vi "7.2-Joystick Server.vi"() -> ()   [LabVIEW 2010]
doc: "Creates a named service and listens on the first available port. Whenever a client connects to the service, it responds with a message containing joystick data. The VI can be stopped using the STOP button."
uses:
  6-OCU Neurons/6.1-UDP Saitek.ctl
  <vilib>/Utility/inputDevices.llb/joystickAcquire.vi
panel:
  out "direction info":T1
  out "button info":T2
  out "axis info":T3
  out "Saitek Controler":T4 {"Right" scale=-32767.0..32767.0; "Left" scale=-32767.0..32767.0; "Yaw" scale=-32767.0..32767.0; "Roll" scale=-32767.0..32767.0; "Pitch" scale=-32767.0..32767.0}
  out "data out":string
  in  "stop":bool
  out "error out":errorcluster
  in  "error in":errorcluster
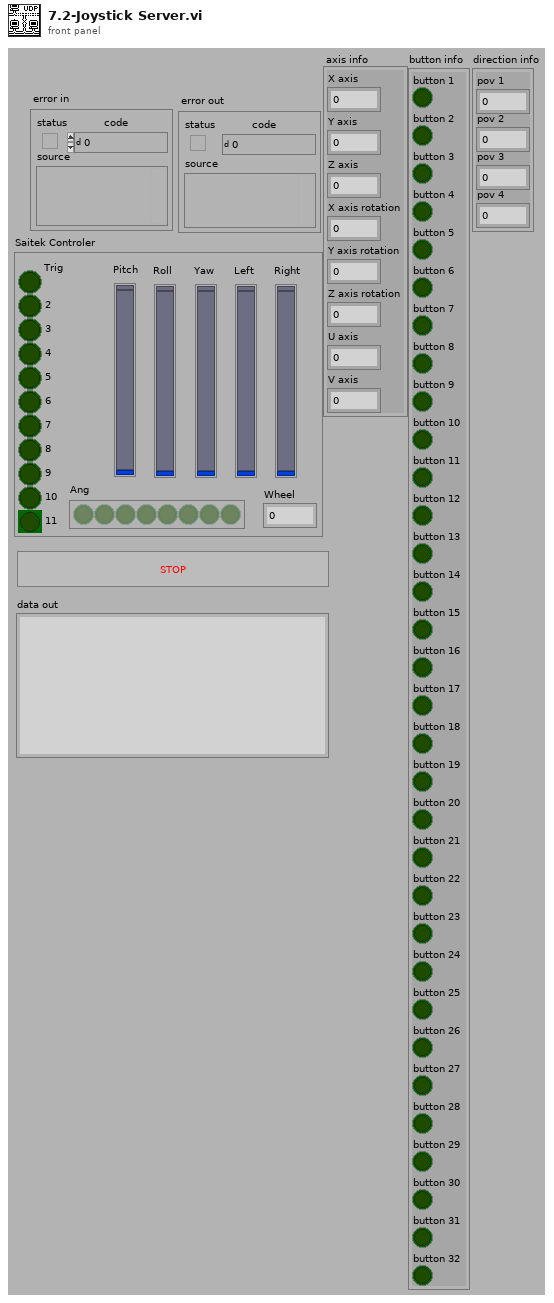
[diagram p1: front panel]
types:
  T1 = cluster{"pov 1":i32, "pov 2":i32, "pov 3":i32, "pov 4":i32}
  T2 = cluster{"button 1":bool, "button 2":bool, "button 3":bool, "button 4":bool, "button 5":bool, "button 6":bool, "button 7":bool, "button 8":bool, "button 9":bool, "button 10":bool, "button 11":bool, "button 12":bool, "button 13":bool, "button 14":bool, "button 15":bool, "button 16":bool, "button 17":bool, "button 18":bool, "button 19":bool, "button 20":bool, "button 21":bool, "button 22":bool, "button 23":bool, "button 24":bool, "button 25":bool, "button 26":bool, "button 27":bool, "button 28":bool, "button 29":bool, "button 30":bool, "button 31":bool, "button 32":bool}
  T3 = cluster{"X axis":i32, "Y axis":i32, "Z axis":i32, "X axis rotation":i32, "Y axis rotation":i32, "Z axis rotation":i32, "U axis":i32, "V axis":i32}
  T4 = typedef "6.1-UDP Saitek.ctl" = cluster{"Trig":bool, "2":bool, "3":bool, "4":bool, "5":bool, "6":bool, "7":bool, "8":bool, "9":bool, "10":bool, "11":bool, "Pitch":i32, "Ang":bool[], "Wheel":dbl, "Roll":i32, "Yaw":i32, "Left":i32, "Right":i32}
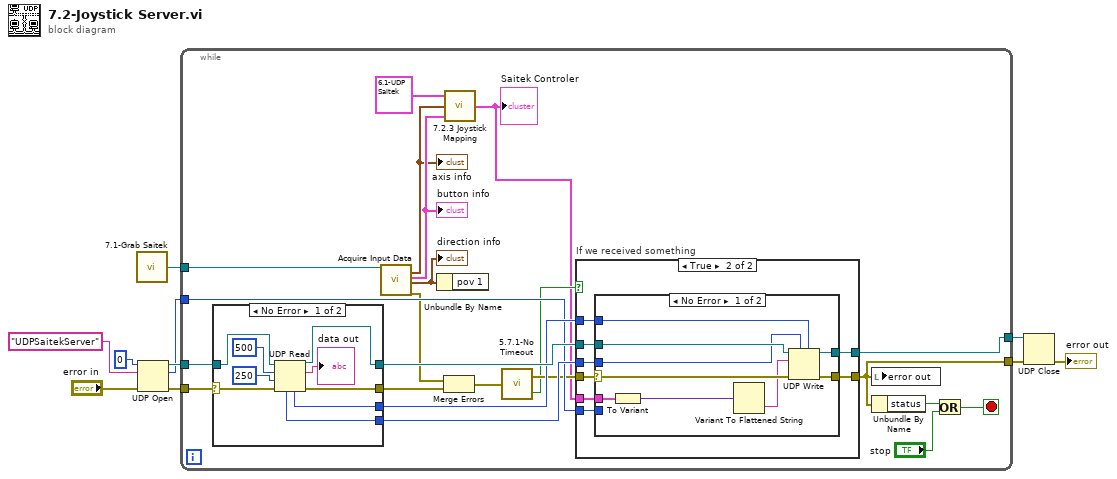
[diagram p0: block diagram]
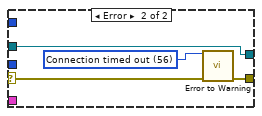
[diagram p3: hidden frame]
diagram:
  n1 = call "7.1-Grab Saitek.vi"() -> ("Saitek ID"=w1:refnum<k1>)
  n2 = UDP Open(8:"error in", 10:"UDPSaitekServer", 11:0) -> (port=w8:refnum<k16>, 0:w7:errorcluster, 2:w3:u16)  [unwired: 2 in]
  n3 = while {
    tunnel: [w20] -> w5
    tunnel: w8 -> [w32]
    tunnel: w7 -> [w29]
    tunnel: [w30] -> w6
    tunnel: w3 -> [w26]
    tunnel: w1 -> [w19]
    stop <- w24 stop-if-true
    n4 = case shown="No Error" w29 {
      selector: w29 -> [w62 w65]
      tunnel: w32 -> [w64 w66]
      tunnel: [w61 w66] -> w31
      tunnel: [w60 w65] -> w18
      tunnel: [w58 _] -> w27
      tunnel: [w59 _] -> w28
      frame No Error {
        n5 = UDP Read(connection ID=w64, max size (548)=500, timeout ms (25000)=250, 8:w62) -> (data out=→"data out":string, error out=w60:errorcluster, 3:w61:refnum<k16>, 4:w58:u16, 6:w59:u32)
      }
      frame Error {
      }
    }
    n6 = call-poly <vilib>:"Acquire Input Data.vi"("device ID"=w19) -> ("axis info"=w12:T3, "button info"=w13:T2, "direction info"=w14:T1, "error out"=w17:errorcluster)  [unwired: 14 in, 1 out]
    "axis info" <- w12
    "button info" <- w13
    "direction info" <- w14
    n7 = Unbundle By Name(w14) -> ()  [unwired: 1 out]
    n8 = Merge Errors(w17, w18) -> (w16:errorcluster)
    n9 = call "7.2.3 Joystick Mapping.vi"("button info"=w13, "axis info"=w12, "Saitek Controler 3"=T4 {"Trig"=FALSE, "2"=FALSE, "3"=FALSE, "4"=FALSE, "5"=FALSE, "6"=FALSE, "7"=FALSE, "8"=FALSE, "9"=FALSE, "10"=FALSE, "11"=FALSE, "Pitch"=0, "Ang"=[], "Wheel"=0.0, "Roll"=0, "Yaw"=0, "Left"=0, "Right"=0} ("Saitek Controler 2")) -> ("Saitek Controler 2"=w11:T4)
    "Saitek Controler" <- w11
    n10 = call "5.7.1-No Timeout.vi"("error in (no error)"=w16) -> ("No Timeout"=w21:bool, "error out"=w22:errorcluster)
    n11 = case "If we received something" shown="True" w21 {
      tunnel: w31 -> [w33 w42]
      tunnel: [w33 w41] -> w30
      tunnel: w28 -> [_ w40]
      tunnel: w27 -> [_ w39]
      tunnel: w26 -> [_ w38]
      tunnel: [w34 w37] -> w20
      tunnel: w22 -> [w34 w36]
      tunnel: w11 -> [_ w35]
      frame False {
      }
      frame True {
        n12 = case shown="No Error" w36 {
          selector: w36 -> [w51 w53]
          tunnel: w42 -> [w48 w55]
          tunnel: [w50 w52] -> w37
          tunnel: [w49 w55] -> w41
          tunnel: w40 -> [w46 _]
          tunnel: w39 -> [w47 _]
          tunnel: w38 -> [_ _]
          tunnel: w35 -> [w43 _]
          frame No Error {
            n13 = To Variant(anything=w43) -> (Variant=w45:variant)
            n14 = Variant To Flattened String(Variant=w45) -> (data string=w44:string)  [unwired: 1 out]
            n15 = UDP Write(address=w46, port or service name=w47, connection ID=w48, data in=w44, 8:w51) -> (error out=w50:errorcluster, 3:w49:refnum<k16>)  [unwired: 1 in]
          }
          frame Error {
            w54 = 56 items=["No Error", "Argument Error", "Memory Full", "Out of Zone", "End of File", "File Already Open", "Generic File IO Error", "File Not Found", "File Permission Error", "Disk Full", "Duplicate Path", "Too Many Files Open", "Not Enabled", "Resource File Not Found", "Cannot Add Resource", "Resource Not Found", "Image Not Found", "Image Memory Error", "Pen Does Not Exist", "Config Bad Type", "Config Token Not Found", "Config Parse Error", "Config Memory Error", "Bad External Code Format", "Bad External Code Offset", "External Code Not Present", "Null Window", "Destroy Window Mixup", "Null Menu", "Print Aborted", "Bad Print Record", "Print Driver Error", "Windows Error During Print", "Memory Error During Print", "Print Dialog Error", "Generic Print Error", "Invalid Device Refnum", "Device Not Found", "Device Parameter Error", "Device Unit Error", "Can't Open Device", "Device Call Aborted", "Generic Error", "Cancelled By User", "Object ID Too Low", "Object ID Too High", "Object Not In Heap", "Unknown Heap", "Bad DefProc ID", "DefProc Not In Table", "Message Out Of Range", "Null Method", "Unknown Message", "Manager Call Not Supported", "Bad address", "Connection In progress", "Connection timed out", "Connection is already in progress", "Network attribute not supported", "Network error", "Address in use", "System out of memory", "Connection aborted", "Connection refused", "Connection is not connected", "Connection is already connected", "Connection closed", "Initialize error (interapplication manager)", "Bad occurrence", "Wait on unbound occurrence handler", "Occurrence queue overflow", "Bad path", "Semaphore not signaled", "Unrecognized type (interapplication manager)"] ("1st Error to Convert")
            n16 = call <vilib>:"Error to Warning.vi"("1st Error to Convert"=w54, "error in"=w53) -> ("warning out"=w52:errorcluster)  [unwired: 13 in]
          }
        }
      }
    }
    n17 = local write "error out"(w20) -> ()
    n18 = Unbundle By Name(w20) -> ("status"=w25:bool)
    n19 = Or(x=w25, y="stop") -> (x .or. y?=w24:bool)
  }
  n20 = UDP Close(connection ID=w6, 8:w5) -> (error out=→"error out":errorcluster)  [unwired: 1 out]
